vi "joystick+conversions.vi"(0 "Refnum in":refnum<k1>, 7 "error in (no error)":errorcluster, 8 "Stop":bool) -> (10 "dir info":i32, 12 "x axis info":i32, 13 "B pressed":bool, 14 "v_radial":dbl, 15 "y axis info":i32, 16 "A pressed":bool, 17 "y axis rot info":i32, 18 "drible":dbl, 19 "v_normal":dbl, 20 "Refnum out":refnum<k1>, 21 "X pressed":bool, 22 "R*w":dbl, 23 "Boolean":bool, 24 "z axis info (drible)":i32, 25 "Y pressed":bool, 26 "x axis rot info":i32, 27 "error out":errorcluster)   [LabVIEW 2016]
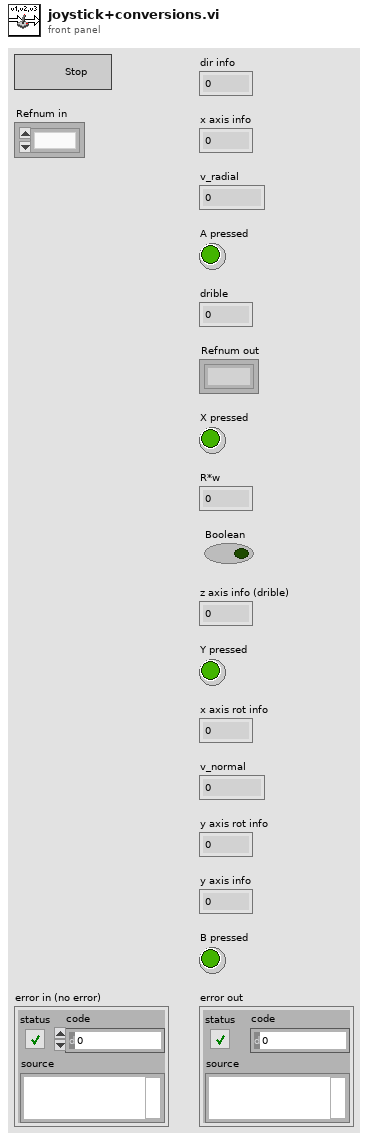
[diagram p1: front panel]
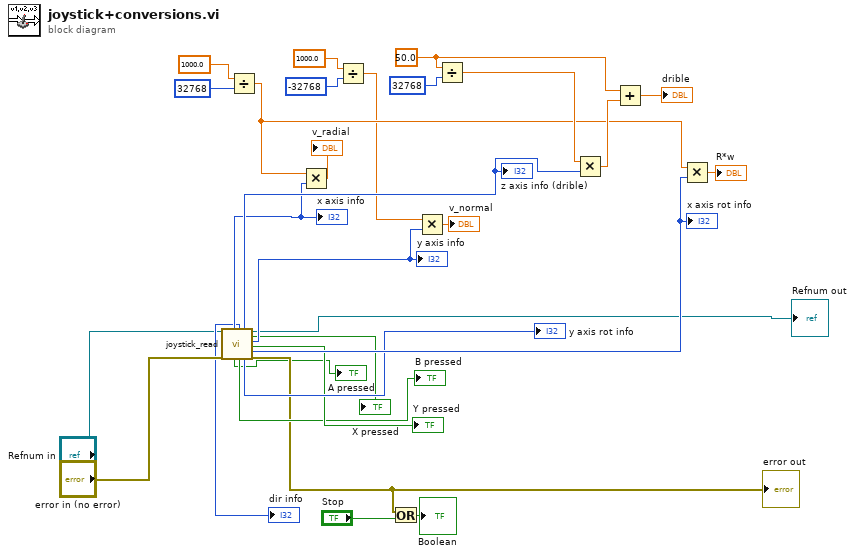
[diagram p0: block diagram]
diagram:
  w30 = 50.0
  n1 = call "joystick_read.vi"("Refnum in"="Refnum in", "error in (no error)"="error in (no error)") -> ("X axis"=w17:i32, "button 1"=→"A pressed":bool, "pov 1"=→"dir info":i32, "button 2"=→"B pressed":bool, "Z axis"=w25:i32, "Y axis rotation"=→"y axis rot info":i32, "Refnum out"=→"Refnum out":refnum<k1>, "button 3"=→"X pressed":bool, "Y axis"=w13:i32, "button 4"=→"Y pressed":bool, "X axis rotation"=w23:i32, "error out"=w7:errorcluster)  [unwired: 6 in]
  "x axis info" <- w17
  "y axis info" <- w13
  "z axis info (drible)" <- w25
  "x axis rot info" <- w23
  "error out" <- w7
  n2 = Divide(x=1000.0, y=32768 ("x")) -> (x/y=w24:dbl)
  n3 = Multiply(x=w24, y=w17) -> (x*y=→"v_radial":dbl)
  n4 = Divide(x=1000.0, y=-32768 ("x")) -> (x/y=w16:dbl)
  n5 = Or(x=w7, y="Stop") -> (x .or. y?=→"Boolean":bool)
  n6 = Multiply(x=w16, y=w13) -> (x*y=→"v_normal":dbl)
  n7 = Divide(x=w30, y=32768 ("x")) -> (x/y=w27:dbl)
  n8 = Multiply(x=w27, y=w25) -> (x*y=w29:dbl)
  n9 = Add(x=w30, y=w29) -> (x+y=→"drible":dbl)
  n10 = Multiply(x=w24, y=w23) -> (x*y=→"R*w":dbl)
